vi "_Object Tester.vi"() -> ()   [LabVIEW 2025, in "Wheatstone Bridge.lvlib" / "Wheatstone Bridge.lvclass"]
uses:
  Wheatstone Bridge.lvclass
  NI-9237/NI-9237.lvclass
  C:/Users/Tyson.Grover/Desktop/Repositories/dqmh-lvoop-template/Libraries/Wheatstone Bridge/Wheatstone Bridge/Wheatstone Bridge.lvclass
  <vilib>/Handler Framework/Handler Framework.lvlib
panel:
  out "error out":errorcluster
  out "Numeric":dbl
  in  "File Path":path
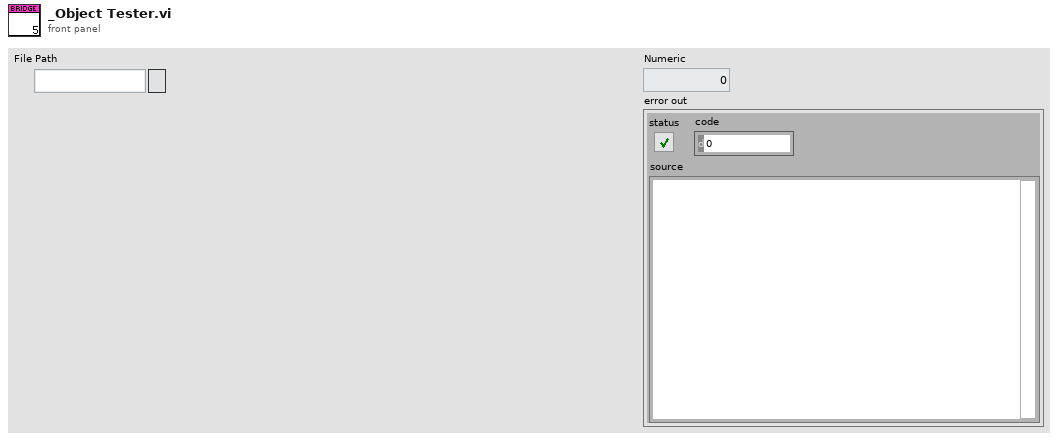
[diagram p1: front panel]
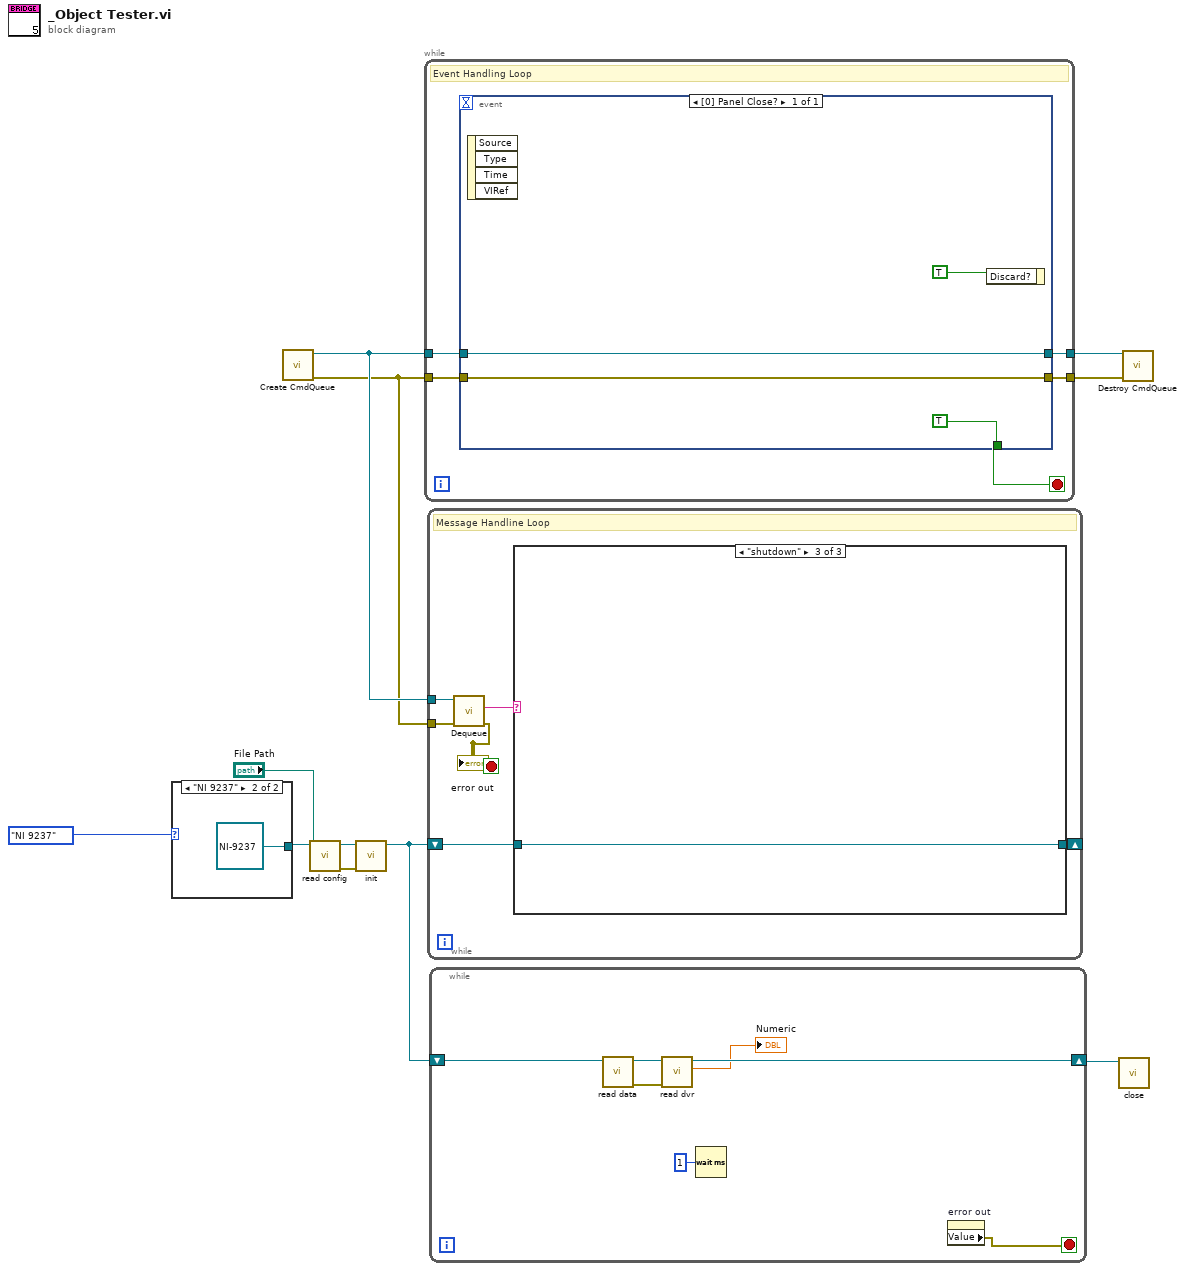
[diagram p0: block diagram]
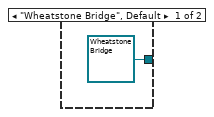
[diagram p2: hidden frame]
diagram:
  n1 = case shown="\"NI 9237\"" enum16{"Wheatstone Bridge", "NI 9237"}."NI 9237" {
    tunnel: [refnum<class "Wheatstone Bridge.lvclass"> refnum ("Wheatstone Bridge.lvlib:Wheatstone Bridge.lvclass") refnum<class "NI-9237.lvclass"> refnum ("Wheatstone Bridge.lvlib:NI-9237.lvclass")] -> w6
    frame "Wheatstone Bridge", Default {
    }
    frame "NI 9237" {
    }
  }
  n2 = call <vilib>:"Create CmdQueue.vi"() -> ("error out"=w10:errorcluster, "CmdQueue out"=w11:refnum<queue>)  [unwired: 10 in]
  n3 = call-dynamic "read config.vi"("File Path"="File Path", "Wheatstone Bridge in"=w6) -> ("error out"=w3:errorcluster, "Wheatstone Bridge out"=w4:refnum<class "Wheatstone Bridge.lvclass">)  [unwired: 8 in]
  n4 = call-dynamic "init.vi"("error in (no error)"=w3, "Wheatstone Bridge in"=w4) -> ("Wheatstone Bridge out"=w2:refnum<class "Wheatstone Bridge.lvclass">)  [unwired: 8 in, 1 out]
  n5 = while {
    tunnel: w11 -> [w17]
    tunnel: w10 -> [w16]
    tunnel: [w15] -> w9
    tunnel: [w14] -> w8
    stop <- w18 stop-if-true
    # "Event Handling Loop"
    n6 = event shown="[0] Panel Close?" {
      selector: _ -> [_]
      dyn-events: _ -> [_]
      timeout: _ -> [_]
      tunnel: [TRUE] -> w18
      tunnel: w17 -> [w20]
      tunnel: w16 -> [w19]
      tunnel: [w20] -> w15
      tunnel: [w19] -> w14
      event Panel Close? {
        n7 = event-data() -> ()  [unwired: 1 in, 4 out]
        n8 = event-data("Discard?"=TRUE) -> ()  [unwired: 1 in, 1 out]
      }
    }
  }
  n9 = while {
    tunnel: w11 -> [w28]
    tunnel: w10 -> [w27]
    shift-right: [w23] -> _
    shift-left: w2 -> [w24]
    stop <- w26 stop-if-true
    # "Message Handline Loop"
    n10 = call <vilib>:"Dequeue.vi"("error in (no error)"=w27, "CmdQueue in"=w28) -> ("error out"=w26:errorcluster, "cmd"=w25:string)  [unwired: 5 in, 3 out]
    "error out" <- w26
    n11 = case shown="\"shutdown\"" w25 {
      tunnel: w24 -> [w29 w30 w31]
      tunnel: [w29 w30 w31] -> w23
      frame Default {
      }
      frame "init" {
      }
      frame "shutdown" {
      }
    }
  }
  n12 = while {
    shift-right: [w35] -> w1
    shift-left: w2 -> [w38]
    stop <- w33 stop-if-true
    n13 = call-dynamic "read data.vi"("Wheatstone Bridge in"=w38) -> ("error out"=w36:errorcluster, "Wheatstone Bridge out"=w37:refnum<class "Wheatstone Bridge.lvclass">)  [unwired: 9 in]
    n14 = call-dynamic "read dvr.vi"("error in (no error)"=w36, "Wheatstone Bridge in"=w37) -> ("Numeric"=→"Numeric":dbl, "Wheatstone Bridge out"=w35:refnum<class "Wheatstone Bridge.lvclass">)  [unwired: 7 in, 1 out]
    n15 = Wait (ms)(milliseconds to wait=u32 1) -> ()  [unwired: 1 out]
    n16 = property on="error out" class="Clust (strict)"() -> ("Value"=w33:errorcluster)  [unwired: 2 in, 2 out]
  }
  n17 = call-dynamic "close.vi"("Wheatstone Bridge in"=w1) -> ()  [unwired: 9 in, 2 out]
  n18 = call <vilib>:"Destroy CmdQueue.vi"("error in (no error)"=w8, "CmdQueue in"=w9) -> ()  [unwired: 9 in, 1 out]
